vi "Get VI Metrics.vi"(8 "error in (no error)":errorcluster, 10 "VI Path":path, 11 "Code Inspector in":refnum<class "Code Inspector Base.lvclass">) -> (0 "error out":errorcluster, 2 "VI Name":string, 3 "Code Inspector out":refnum<class "Code Inspector Base.lvclass">, 4 "Total Diagram Count":i32, 5 "Total Node Count":i32, 6 "Uncovered Diagram Count":i32, 7 "Uncovered Node Count":i32)   [LabVIEW 2017, in "Cobertura.lvlib" / "Code Inspector Base.lvclass"]
uses:
  Code Inspector Base.lvclass
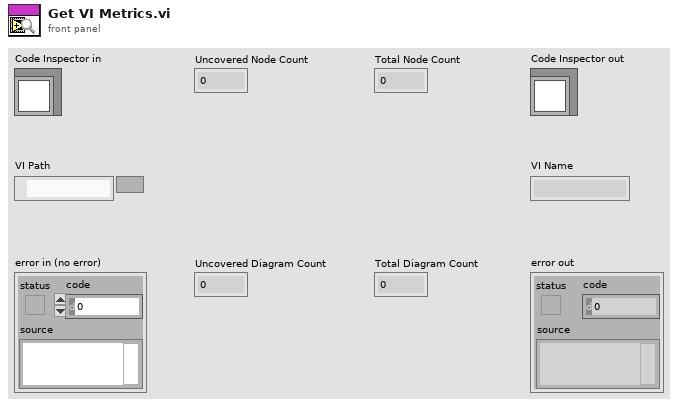
[diagram p1: front panel]
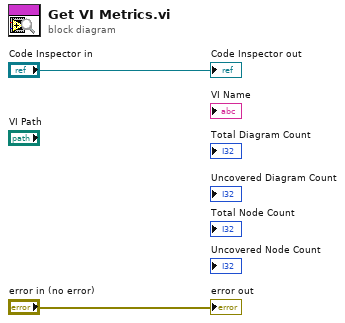
[diagram p0: block diagram]
diagram:
  "error out" <- "error in (no error)"
  "Code Inspector out" <- "Code Inspector in"
